vi "XY Graph Show-Hide Grid.vi"(4 "# Y Scales (1)":i32=1, 6 "# X Scales (1)":i32=1, 8 "Error In":errorcluster, 9 "Hide (F) /Show (T)":bool, 11 "XY Graph Ref":T1) -> (0 "Error Out":errorcluster, 1 "Grid Shown?":bool)   [LabVIEW 2019, in "XY Graph Add-Ons.lvlib"]
uses:
  XY Graph Add-Ons.lvlib
  XY Graph Refnum.ctl
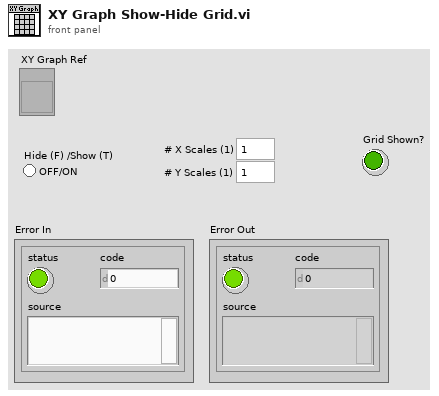
[diagram p1: front panel]
types:
  T1 = typedef "XY Graph Add-Ons.lvlib/XY Graph Refnum.ctl" = refnum<vi>
  T2 = typedef "LVMajorAndMinorColorsTypeDef.ctl" = cluster{"Major Color":u32, "Minor Color":u32}
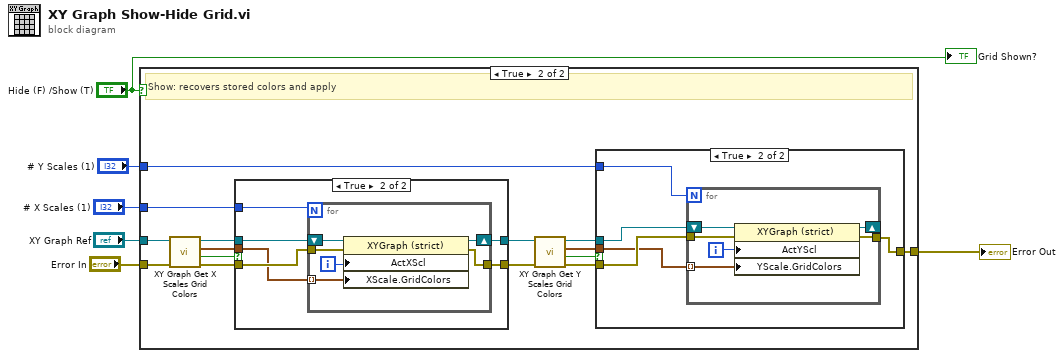
[diagram p0: block diagram]
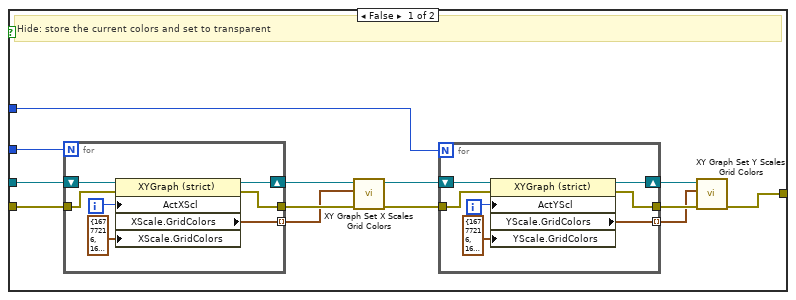
[diagram p2: hidden frame]
diagram:
  n1 = case shown="True" "Hide (F) /Show (T)" {
    tunnel: "XY Graph Ref" -> [w19 w46]
    tunnel: "Error In" -> [w18 w43]
    tunnel: [w7 w44] -> w2
    tunnel: "# X Scales (1)" -> [w15 w47]
    tunnel: "# Y Scales (1)" -> [w14 w45]
    frame False {
      # "Hide: store the current colors and set to transparent"
      n2 = for {
        N: w15 -> [_]
        tunnel: [w29] -> w16 mode=indexing
        shift-right: [w30] -> w12
        shift-left: w19 -> [w33]
        tunnel: w18 -> [w32]
        tunnel: [w31] -> w17
        i -> [w27]
        n3 = property class="XYGraph (strict)"(reference=w33, error in=w32, "ActXScl"=w27, "XScale.GridColors"=cluster{"Major Color":u32, "Minor Color":u32} {"Major Color"=16777216, "Minor Color"=16777216} ("X Scale.Grid Colors")) -> (reference out=w30:T1, error out=w31:errorcluster, "XScale.GridColors"=w29:T2)
      }
      n4 = call "XY Graph Set X Scales Grid Colors.vi"("error in (no error)"=w17, "Array of Grid Colors"=w16, "XYGraph in"=w12) -> ("error out"=w13:errorcluster, "XYGraph out"=w11:T1)  [unwired: 7 in]
      n5 = for {
        N: w14 -> [_]
        tunnel: [w22] -> w8 mode=indexing
        shift-right: [w23] -> w10
        shift-left: w11 -> [w26]
        tunnel: w13 -> [w25]
        tunnel: [w24] -> w9
        i -> [w20]
        n6 = property class="XYGraph (strict)"(reference=w26, error in=w25, "ActYScl"=w20, "YScale.GridColors"=cluster{"Major Color":u32, "Minor Color":u32} {"Major Color"=16777216, "Minor Color"=16777216} ("X Scale.Grid Colors")) -> (reference out=w23:T1, error out=w24:errorcluster, "YScale.GridColors"=w22:T2)
      }
      n7 = call "XY Graph Set Y Scales Grid Colors.vi"("error in (no error)"=w9, "Array of Grid Colors"=w8, "XYGraph in"=w10) -> ("error out"=w7:errorcluster)  [unwired: 7 in, 1 out]
    }
    frame True {
      # "Show: recovers stored colors and apply"
      n8 = call "XY Graph Get X Scales Grid Colors.vi"("error in (no error)"=w43, "XYGraph in"=w46) -> ("error out"=w48:errorcluster, "Was Tag Found?"=w42:bool, "X Scale.Grid Colors"=w40:cluster{"Major Color":u32, "Minor Color":u32}[], "XYGraph out"=w41:T1)  [unwired: 6 in]
      n9 = case shown="True" w42 {
        tunnel: w40 -> [_ w63]
        tunnel: w48 -> [w61 w64]
        tunnel: w47 -> [_ w68]
        tunnel: w41 -> [w62 w67]
        tunnel: [w62 w66] -> w38
        tunnel: [w61 w65] -> w39
        frame False {
        }
        frame True {
          n10 = for {
            N: w68 -> [_]
            shift-right: [w72] -> w66
            shift-left: w67 -> [w74]
            tunnel: [w73] -> w65
            tunnel: w64 -> [w71]
            tunnel: w63 -> [w70] mode=indexing
            i -> [w69]
            n11 = property class="XYGraph (strict)"(reference=w74, error in=w71, "ActXScl"=w69, "XScale.GridColors"=w70) -> (reference out=w72:T1, error out=w73:errorcluster)
          }
        }
      }
      n12 = call "XY Graph Get Y Scales Grid Colors.vi"("error in (no error)"=w39, "XYGraph in"=w38) -> ("error out"=w37:errorcluster, "Was Tag Found?"=w35:bool, "Y Scale.Grid Colors"=w34:cluster{"Major Color":u32, "Minor Color":u32}[], "XYGraph out"=w36:T1)  [unwired: 6 in]
      n13 = case shown="True" w35 {
        tunnel: w45 -> [_ w54]
        tunnel: [w49 w53] -> w44
        tunnel: w37 -> [w49 w52]
        tunnel: w36 -> [_ w51]
        tunnel: w34 -> [_ w50]
        frame False {
        }
        frame True {
          n14 = for {
            N: w54 -> [_]
            shift-right: [w58] -> _
            shift-left: w51 -> [w60]
            tunnel: [w59] -> w53
            tunnel: w52 -> [w57]
            tunnel: w50 -> [w56] mode=indexing
            i -> [w55]
            n15 = property class="XYGraph (strict)"(reference=w60, error in=w57, "ActYScl"=w55, "YScale.GridColors"=w56) -> (reference out=w58:T1, error out=w59:errorcluster)
          }
        }
      }
    }
  }
  "Error Out" <- w2
  "Grid Shown?" <- "Hide (F) /Show (T)"
